vi "Global Reset.vi"(8 "error in":errorcluster, 11 "Clobal Reset":refnum<vi>) -> (0 "error out":errorcluster)   [LabVIEW 2023, in "GUI.lvlib" / "Diagnostic.lvlib" / "Diagnostic.lvclass"]
uses:
  Diagnostic.lvclass
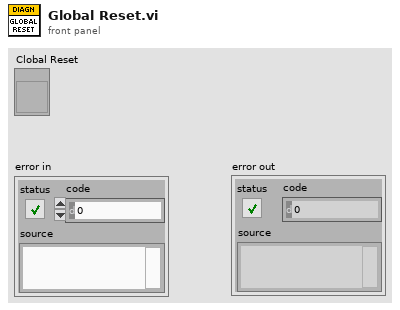
[diagram p1: front panel]
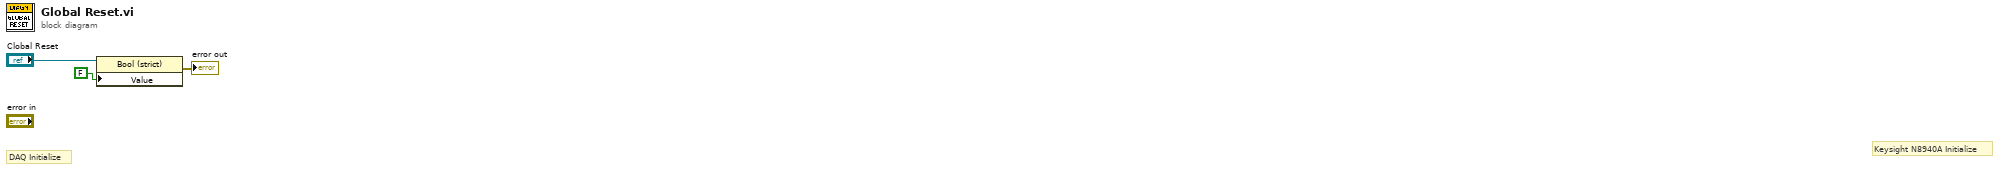
[diagram p0: block diagram]
diagram:
  # "Keysight N8940A Initialize"
  # "DAQ Initialize"
  n1 = property class="Bool (strict)"(reference="Clobal Reset", "Value"=FALSE) -> (error out=→"error out":errorcluster)  [unwired: 1 in, 1 out]
